vi "Auto_Conf.vi"() -> ()   [LabVIEW 2011]
panel:
  in  "Automodes":string[](array[string])=["none.bee", "auto_key_center_bridge_roll.bee", "auto_side_bridge_nofire.bee", "auto_side_bridge.bee", "auto_key_center_bridge_first.bee", "auto_key_center_bridge_prealign.bee", "auto_key_center_key_stay.bee", "auto_key_front_drive.bee", "auto_key_center_bridge_nofire.bee", "auto_key_center_bridge_first_four.bee"]
  in  "hdg target":dbl
  in  "Verbose Debug Mode (Dangerous?)":bool
  in  "AutoToRun":u8
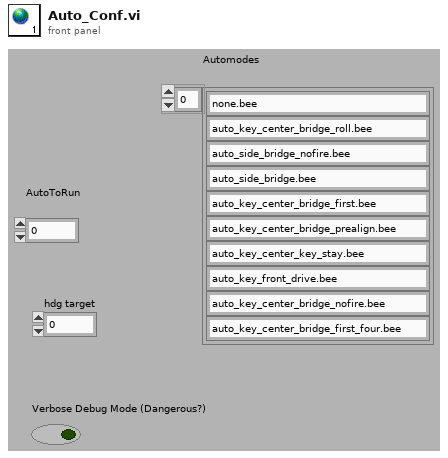
[diagram p1: front panel]
diagram:
